vi "PV Establish Connection.vi"(6 "Access (R/W allowed)":T1, 7 "Mode (buffer)":u16(ring)=1 items=["commit", "buffer"], 8 "Error In":errorcluster, 11 "PVConnections in":refnum<class "PVConnection.lvclass">[](array[class])) -> (0 "Error Out":errorcluster, 3 "PVConnections out":refnum<class "PVConnection.lvclass">[](array[class]))   [LabVIEW 2016, in "CS++Utilities.lvlib"]
doc: "Connect PV. In case of DSC the last PV will commit."
uses:
  CS++Utilities.lvlib
  Classes/CS++ProcessVariables/PVConnection/PVConnection.lvclass
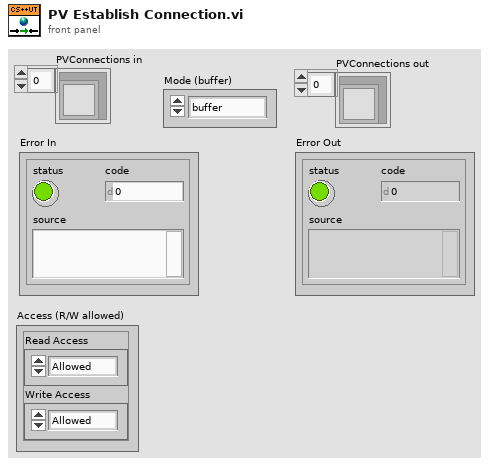
[diagram p1: front panel]
types:
  T1 = cluster{"Read Access":enum8{"Allowed", "Required", "None"}, "Write Access":enum8{"Allowed", "Required", "None"}}
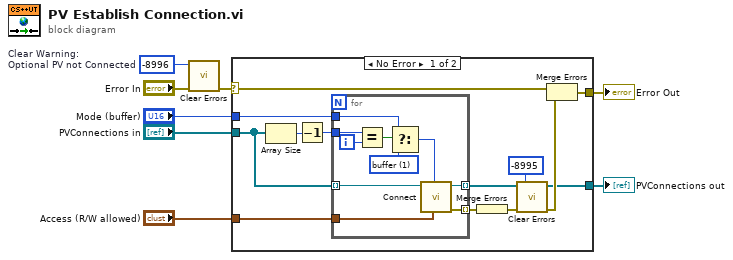
[diagram p0: block diagram]
diagram:
  w6 = -8996  # Clear Warning: Optional PV not Connected
  n1 = call <vilib>:"Clear Errors.vi"("error in (no error)"="Error In", "specific error code to clear (0: all)"=w6) -> ("error out"=w7:errorcluster)  [unwired: 4 in, 1 out]
  n2 = case shown="No Error" w7 {
    selector: w7 -> [w20 w31]
    tunnel: "PVConnections in" -> [w12 w32]
    tunnel: [w19 w31] -> w8
    tunnel: [w11 w32] -> w3
    tunnel: "Access (R/W allowed)" -> [w10 _]
    tunnel: "Mode (buffer)" -> [w9 _]
    frame No Error {
      n3 = Array Size(array=w12) -> (size(s)=w15:i32)
      n4 = Decrement(x=w15) -> (x-1=w14:i32)
      n5 = for {
        tunnel: w12 -> [w30] mode=indexing
        tunnel: [w29] -> w11 mode=indexing
        tunnel: w10 -> [w28]
        tunnel: [w27] -> w16 mode=indexing
        tunnel: w14 -> [w22]
        tunnel: w9 -> [w21]
        i -> [w23]
        w25 = u16 1 items=["commit", "buffer"] ("Mode (commit)")
        n6 = Equal?(x=w22, y=w23) -> (x = y?=w26:bool)
        n7 = Select(t=w21, s=w26, f=w25) -> (s? t:f=w24:u16)
        n8 = call "Connect.vi"("Access (R/W allowed)"=w28, "Mode (buffer)"=w24, "PVConnection in"=w30) -> ("Error Out"=w27:errorcluster, "PVConnection out"=w29:refnum<class "PVConnection.lvclass">)  [unwired: 7 in]
      }
      n9 = Merge Errors(w16) -> (w13:errorcluster)
      n10 = call <vilib>:"Clear Errors.vi"("error in (no error)"=w13, "specific error code to clear (0: all)"=-8995) -> ("error out"=w18:errorcluster)  [unwired: 4 in, 1 out]
      n11 = Merge Errors(w20, w18) -> (w19:errorcluster)
    }
    frame Error {
    }
  }
  "Error Out" <- w8
  "PVConnections out" <- w3
